vi "ComboBox.vi"() -> ()   [LabVIEW 2018]
panel:
  out "String":string
  in  "Combo Box":string(combo)="Sunday"
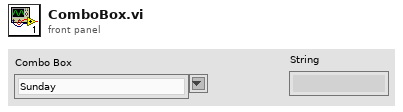
[diagram p1: front panel]
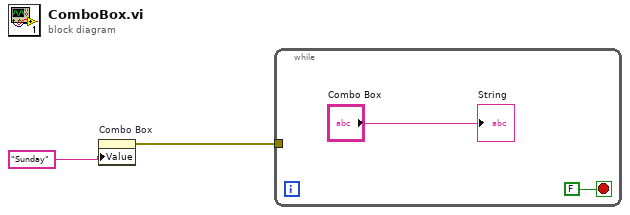
[diagram p0: block diagram]
diagram:
  n1 = property on="Combo Box" class="CmbBox"("Value"="Sunday") -> (error out=w2:errorcluster)  [unwired: 2 in, 1 out]
  n2 = while {
    tunnel: w2 -> [_]
    stop <- FALSE stop-if-true
    "String" <- "Combo Box"
  }
